vi "UDP Test.vi"() -> ()   [LabVIEW 2025]
panel:
  out "value":T1
  in  "output cluster":T1
  out "error out":errorcluster
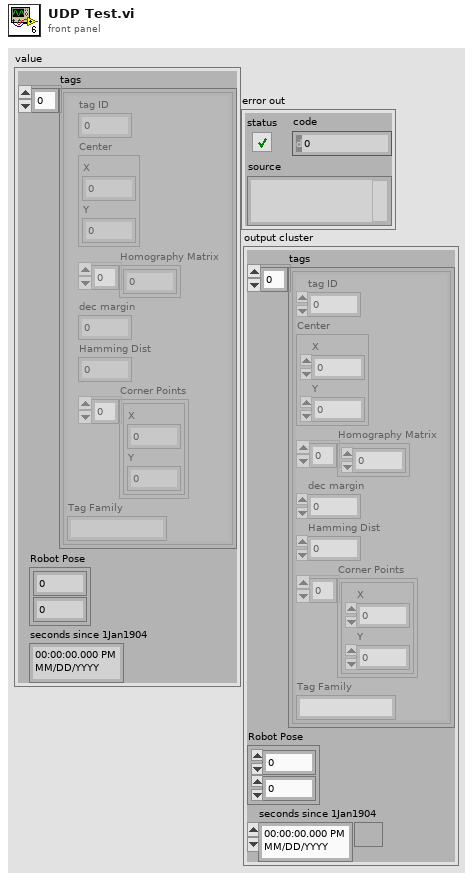
[diagram p1: front panel]
types:
  T1 = cluster{"tags":cluster{"tag ID":i32, "Center":cluster{"X":dbl, "Y":dbl}, "Homography Matrix":dbl[], "dec margin":dbl, "Hamming Dist":i32, "Corner Points":cluster{"X":dbl, "Y":dbl}[], "Tag Family":string}[], "Robot Pose":cluster{dbl, dbl}, "seconds since 1Jan1904":timestamp}
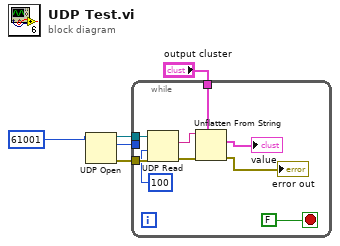
[diagram p0: block diagram]
diagram:
  n1 = UDP Open(11:u16 61001 ("port")) -> (port=w2:refnum<k16>, 0:w4:errorcluster, 2:w3:u16)  [unwired: 4 in]
  n2 = while {
    tunnel: w4 -> [w14]
    tunnel: w3 -> [_]
    tunnel: w2 -> [w13]
    tunnel: "output cluster" -> [w10]
    stop <- FALSE stop-if-true
    n3 = UDP Read(connection ID=w13, timeout ms (25000)=100, 8:w14) -> (data out=w9:string, error out=w7:errorcluster)  [unwired: 1 in, 3 out]
    n4 = Unflatten From String(type=w10, binary string=w9, error in (no error)=w7) -> (value=→"value":T1, error out=→"error out":errorcluster)  [unwired: 2 in, 1 out]
  }
